vi "Automation - Run Stimulus Profile.vi"() -> ()   [LabVIEW 2010]
doc: "Sample numeric display item."
uses:
  <vilib>/NI VeriStand/Display Template Support/Display Template Support.llb/cluster_Screen Item Settings.ctl
  <vilib>/NI VeriStand/Display Template Support/Display Template Support.llb/cluster_Graph Scale Settings.ctl
  <vilib>/NI VeriStand/Display Template Support/Display Template Support.llb/cluster_Graph Plot Settings.ctl
  <vilib>/NI VeriStand/Display Template Support/Display Template Support.llb/enum_Display Template Handler Minimal To Widget Msg.ctl
  <vilib>/NI VeriStand/Display Template Support/Display Template Support.llb/enum_Display Template Handler Minimal To Workspace.ctl
  <vilib>/NI VeriStand/Display Template Support/Display Template Support.llb/sub_Display Template Handler Custom.vi
  <vilib>/NI Veristand/Execution/Stimulus/NI_VS Stimulus ExecutionAPI.lvlib
panel:
  in  "NIVS.Gateway IP Address":string
  out "Error":bool
  out "Logging Base Path":string
  in  "Profiles":u16(ring)
  in  "Stop":bool
  in  "RUN":bool
  out "Stimulus Profile Base Path":string
  in  "Item.Data":T1
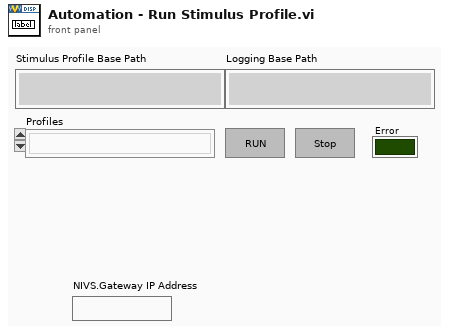
[diagram p1: front panel]
types:
  T1 = typedef "cluster_Screen Item Settings.ctl" = cluster{"Template VI":string, "Position X":i32, "Position Y":i32, "Custom":string, "Show Title Bar":bool, "ID":i32, "Always On Top":bool, "Allow Resize":bool, "Allow Minimize":bool, "Allow Close":bool, "Size to Screen":bool, "Screen.ID":i32, "State":enum16{"Normal", "New"}, "Title":string, "Window Bounds":cluster{"[0]":i16, "[1]":i16, "[2]":i16, "[3]":i16}, "Channel Ref":u64, "Unit":string, "Default Units?":bool, "Flash Limit?":bool, "Color 1":u32, "Color 2":u32, "Color 3":u32, "Color 4":u32, "Bck Color":u32, "Fore Color":u32, "Limit 1":dbl, "Limit 2":dbl, "Limit 3":dbl, "Limit 4":dbl, "Limit Mode 1":i32, "Limit Mode 2":i32, "Limit Mode 3":i32, "Limit Mode 4":i32, "Scale Precision":i32, "Scale Min":dbl, "Scale Max":dbl, "Format":i32, "Precision":i32, "Background Type":i32, "IDs":i32[], "Units":string[], "Labels":string[], "Scale Factor":dbl, "Scale Offset":dbl, "YScale Index":u32[], "XScale":T2, "YScales":T2[], "Plots":T3[], "Update Period":dbl, "History Length":dbl, "My.Ref":refnum<vi>, "Is Control?":bool, "Channel Paths":string[], "Custom Data":variant}
  T2 = typedef "cluster_Graph Scale Settings.ctl" = cluster{"Format":u8, "Precision":u8, "Fit":u8, "Label":string, "Use Default Label":bool, "Label Visible":bool, "Min":dbl, "Max":dbl}
  T3 = typedef "cluster_Graph Plot Settings.ctl" = cluster{"Bar Style":u8, "Fill To":i16, "Fill/PtColor":u32, "Line Style":u8, "Line Width":u8, "Color":u32, "Interp":u8, "Point Style":u8}
  T4 = cluster{"Stimulus Profiles Base Path Folder Out":path, "Logging Base Path Folder Out":path}
  T5 = typedef "enum_Display Template Handler Minimal To Workspace.ctl" = cluster{"Operation":enum16{"SetCustomData", "DeleteItem"}, "Data":variant}
  T6 = typedef "enum_Display Template Handler Minimal To Widget Msg.ctl" = enum16{"Stop", "LaunchConfigDialog"}
  T7 = typedef "NI_VS Stimulus ExecutionAPI.lvlib/StimulusAPI.ctl" = refnum<k24>
  T8 = cluster{"Stimulus Profiles Base Path Folder Out":path, "Paths Out":path[], "Logging Base Path Folder Out":path}
  T9 = enum8{"Enabled", "Disabled", "Disabled and Grayed Out"}
  T10 = cluster{"Stimulus Profiles Base Path Folder Out":path, "Stimulus Profiles Logging Base Path Folder Out":path}
  T11 = cluster{"Stimulus Profiles Base Path Folder Out":path, "Paths Out":path[], "Stimulus Profiles Logging Base Path Folder Out":path}
  T12 = typedef "NI_VS Stimulus ExecutionAPI.lvlib/StimulusState.ctl" = enum16{"Stopped", "Starting", "Running", "Stopping"}
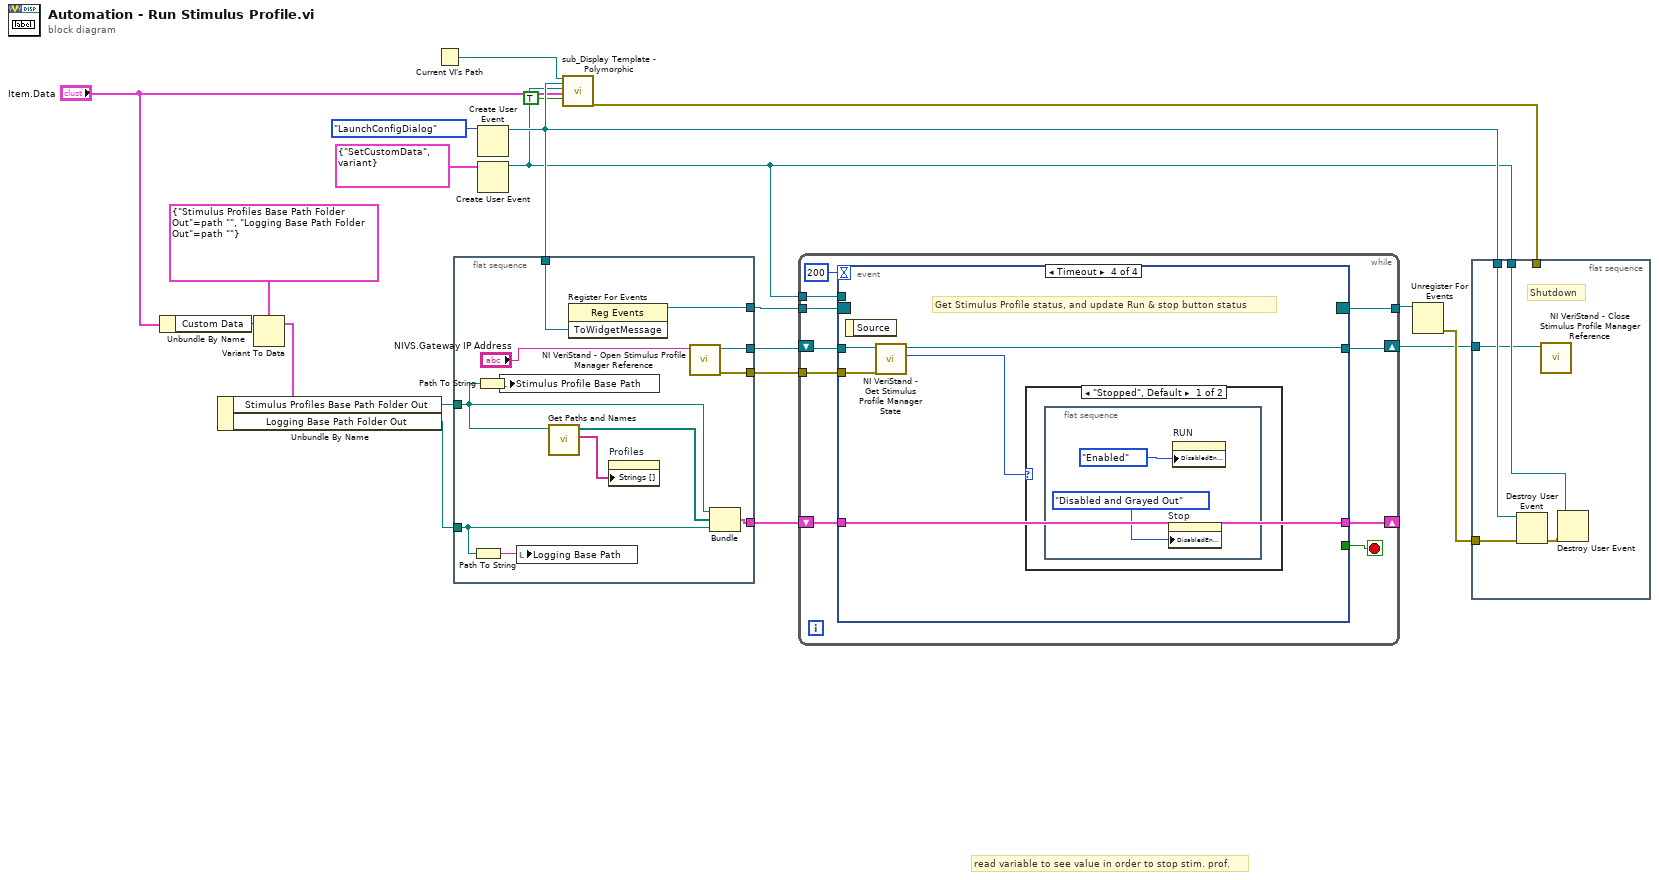
[diagram p0: block diagram]
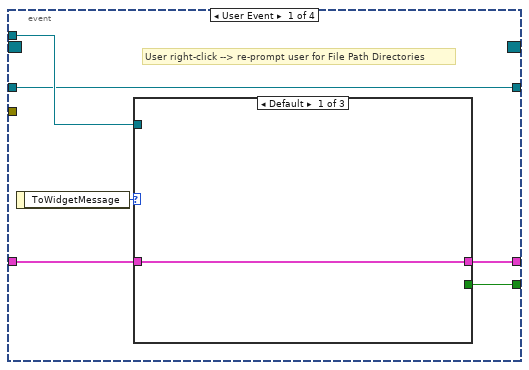
[diagram p2: hidden frame]
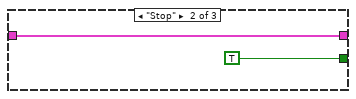
[diagram p3: hidden frame]
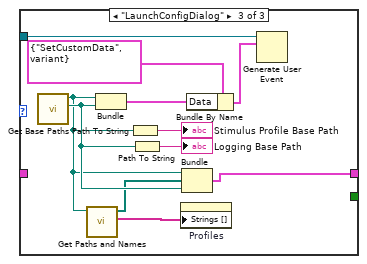
[diagram p4: hidden frame]
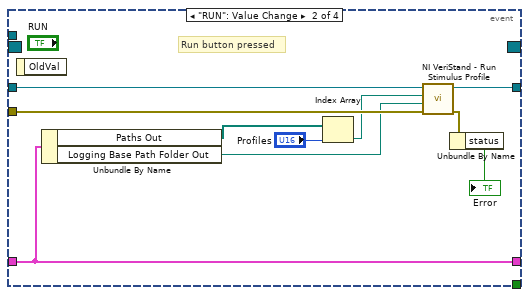
[diagram p5: hidden frame]
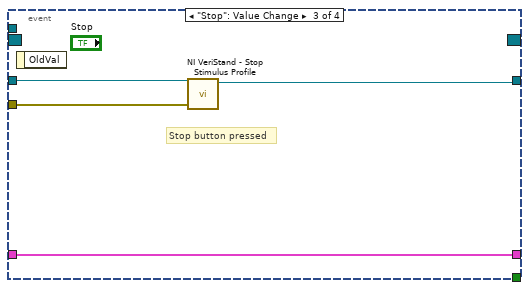
[diagram p6: hidden frame]
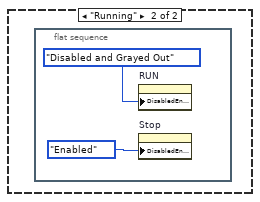
[diagram p7: hidden frame]
diagram:
  # "read variable to see value in order to stop stim. prof."
  n1 = Unbundle By Name("Item.Data") -> ("Custom Data"=w8:variant)
  n2 = Variant To Data(Variant=w8, type=T4 {"Stimulus Profiles Base Path Folder Out"=path "", "Logging Base Path Folder Out"=path ""}) -> (data=w7:T4)  [unwired: 1 in, 1 out]
  n3 = Unbundle By Name(w7) -> ("Stimulus Profiles Base Path Folder Out"=w4:path, "Logging Base Path Folder Out"=w3:path)
  n4 = Current VI's Path() -> (path=w13:path)
  n5 = flat-sequence {
    tunnel: [w32] -> w18
    tunnel: w15 -> [w31]
    tunnel: [w30] -> w10
    tunnel: w4 -> [w24]
    tunnel: [w28] -> w1
    tunnel: w3 -> [w22]
    tunnel: [w25] -> w2
    frame #0 {
      n6 = Path To String(path=w22) -> (string=w26:string)
      n7 = Path To String(path=w24) -> (string=w27:string)
      n8 = local write "Stimulus Profile Base Path"(w27) -> ()
      n9 = local write "Logging Base Path"(w26) -> ()
      n10 = call "Get Paths and Names.vi"("Stimulus Profiles Base Path Folder"=w24) -> ("Profile Names Out"=w29:string[], "Paths Out"=w23:path[])  [unwired: 9 in]
      n11 = register-events(w31) -> (reference out=w32:refnum<event-registration>)  [unwired: 2 in, 1 out]
      n12 = property on="Profiles" class="Ring (strict)"("Strings []"=w29) -> ()  [unwired: 2 in, 2 out]
      n13 = call <vilib>:"NI VeriStand - Open Stimulus Profile Manager Reference.vi"("Gateway IP Address (\"\": localhost)"="NIVS.Gateway IP Address") -> ("error out"=w28:errorcluster, "StimulusProfileManager"=w30:T7)  [unwired: 9 in]
      n14 = Bundle("Stimulus Profiles Base Path Folder Out"=w24, "Paths Out"=w23, "Logging Base Path Folder Out"=w22) -> (w25:T8)  [unwired: 1 in]
    }
  }
  n15 = Create User Event(user event datatype=enum_Display_Template_Handler_Minimal_To_Widget_Msg."LaunchConfigDialog" ("ToWidgetMessage")) -> (user event=w15:refnum<user-event>)  [unwired: 1 in, 1 out]
  n16 = Create User Event(user event datatype=T5 {"Operation"=enum."SetCustomData", "Data"=variant} ("Data")) -> (user event=w12:refnum<user-event>)  [unwired: 1 in, 1 out]
  n17 = call-poly <vilib>:"sub_Display Template - Polymorphic.vi"("Parent.Path"=w13, "ToWidgetEvent"=w15, "ToWorkspace"=w12, "Item.Data"="Item.Data", "Resizable"=TRUE) -> ("error out"=w20:errorcluster)  [unwired: 1 in, 13 out]
  n18 = while {
    tunnel: w18 -> [w42]
    tunnel: [w40] -> w17
    tunnel: w12 -> [w39]
    shift-right: [w37] -> w9
    shift-left: w10 -> [w38]
    shift-right: [w35] -> _
    shift-left: w2 -> [w34]
    tunnel: w1 -> [w33]
    stop <- w41 stop-if-true
    n19 = event shown="[3] Timeout" {
      selector: w42 -> [_ _ _ _]
      dyn-events: [_ _ _ _] -> w40
      timeout: 200 -> [_ _ _ _]
      tunnel: [w47 _ _ _] -> w41
      tunnel: w39 -> [w46 _ _ _]
      tunnel: w38 -> [w45 w72 w76 w81]
      tunnel: [w45 w71 w75 w80] -> w37
      tunnel: w33 -> [_ w70 w74 w78]
      tunnel: [w44 w65 w73 w77] -> w35
      tunnel: w34 -> [w43 w65 w73 w77]
      event User Event {
        # "User right-click --> re-prompt user for File Path Directories"
        n20 = event-data() -> ("ToWidgetMessage"=w48:T6)  [unwired: 1 out]
        n21 = case shown="Default" w48 {
          tunnel: [_ TRUE _] -> w47
          tunnel: w46 -> [_ _ w62]
          tunnel: [w49 w50 w54] -> w44
          tunnel: w43 -> [w49 w50 _]
          frame Default {
          }
          frame "Stop" {
          }
          frame "LaunchConfigDialog" {
            n22 = call "Get Base Paths.vi"() -> ("Stimulus Profiles Logging Base Path Folder Out"=w56:path, "Stimulus Profiles Base Path Folder Out"=w53:path)  [unwired: 10 in]
            n23 = call "Get Paths and Names.vi"("Stimulus Profiles Base Path Folder"=w53) -> ("Profile Names Out"=w61:string[], "Paths Out"=w55:path[])  [unwired: 9 in]
            n24 = Bundle("Stimulus Profiles Base Path Folder Out"=w53, "Stimulus Profiles Logging Base Path Folder Out"=w56) -> (w52:T10)  [unwired: 1 in]
            n25 = Path To String(path=w53) -> (string=→"Stimulus Profile Base Path":string)
            n26 = Path To String(path=w56) -> (string=→"Logging Base Path":string)
            n27 = property on="Profiles" class="Ring (strict)"("Strings []"=w61) -> ()  [unwired: 2 in, 2 out]
            n28 = Bundle("Stimulus Profiles Base Path Folder Out"=w53, "Paths Out"=w55, "Stimulus Profiles Logging Base Path Folder Out"=w56) -> (w54:T11)  [unwired: 1 in]
            n29 = Bundle By Name(cluster=T5 {"Operation"=enum."SetCustomData", "Data"=variant} ("event data"), "Data"=w52) -> (w59:T5)
            n30 = Generate User Event(user event=w62, event data cluster=w59) -> ()  [unwired: 1 in, 2 out]
          }
        }
      }
      event "RUN": Value Change {
        # "Run button pressed"
        n31 = event-data() -> ()  [unwired: 2 out]
        n32 = Unbundle By Name(w65) -> ("Paths Out"=w67:path[], "Logging Base Path Folder Out"=w66:path)
        n33 = Index Array(array=w67, index="Profiles") -> (element=w68:path)
        n34 = call <vilib>:"NI VeriStand - Run Stimulus Profile.vi"("error in (no error)"=w70, "Logging Directory Base Path"=w66, "Stimulus Profile File"=w68, "StimulusProfileManager in"=w72) -> ("error out"=w64:errorcluster, "StimulusProfileManager out"=w71:T7)  [unwired: 6 in]
        n35 = Unbundle By Name(w64) -> ("status"=→"Error":bool)
      }
      event "Stop": Value Change {
        # "Stop button pressed"
        n36 = event-data() -> ()  [unwired: 2 out]
        n37 = call <vilib>:"NI VeriStand - Stop Stimulus Profile.vi"("error in (no error)"=w74, "StimulusProfileManager in"=w76) -> ("StimulusProfileManager out"=w75:T7)  [unwired: 8 in, 1 out]
      }
      event Timeout {
        # "Get Stimulus Profile status, and update Run & stop button status"
        n38 = event-data() -> ()  [unwired: 2 out]
        n39 = call <vilib>:"NI VeriStand - Get Stimulus Profile Manager State.vi"("error in (no error)"=w78, "StimulusProfileManager in"=w81) -> ("State"=w79:T12, "StimulusProfileManager out"=w80:T7)  [unwired: 7 in, 1 out]
        n40 = case shown="\"Stopped\", Default" w79 {
          frame "Stopped", Default {
            n41 = flat-sequence {
              frame #0 {
                n42 = property on="Stop" class="Bool"("DisabledEnum"=T9."Disabled and Grayed Out" ("Disabled")) -> ()  [unwired: 2 in, 2 out]
                n43 = property on="RUN" class="Bool"("DisabledEnum"=T9."Enabled" ("Disabled")) -> ()  [unwired: 2 in, 2 out]
              }
            }
          }
          frame "Running" {
            n44 = flat-sequence {
              frame #0 {
                n45 = property on="RUN" class="Bool"("DisabledEnum"=T9."Disabled and Grayed Out" ("Disabled")) -> ()  [unwired: 2 in, 2 out]
                n46 = property on="Stop" class="Bool"("DisabledEnum"=T9."Enabled" ("Disabled")) -> ()  [unwired: 2 in, 2 out]
              }
            }
          }
        }
      }
    }
  }
  n47 = Unregister For Events(event registration refnum=w17) -> (error out=w16:errorcluster)  [unwired: 1 in]
  n48 = flat-sequence {
    tunnel: w20 -> [_]
    tunnel: w16 -> [w89]
    tunnel: w15 -> [w90]
    tunnel: w12 -> [w87]
    tunnel: w9 -> [w86]
    frame #0 {
      # "Shutdown"
      n49 = Destroy User Event(user event=w90, error in=w89) -> (error out=w88:errorcluster)
      n50 = call <vilib>:"NI VeriStand - Close Stimulus Profile Manager Reference.vi"("StimulusProfileManager"=w86) -> ()  [unwired: 10 in, 1 out]
      n51 = Destroy User Event(user event=w87, error in=w88) -> ()  [unwired: 1 out]
    }
  }
